vi "wrap.GetNameList.vi"(0 "class.GLue in":refnum<class "class.GLue.lvclass">, 5 "length":i32, 9 "index":i32=-1, 11 "error in (no error)":errorcluster, 13 "StringArray in":string[][](array[string])) -> (4 "class.GLue out":refnum<class "class.GLue.lvclass">, 6 "StringArray out":string[][](array[string]), 10 "return":i32, 15 "error out":errorcluster)   [LabVIEW 2014, in "GLue.lvlib" / "class.GLue.lvclass"]
uses:
  class.GLue.lvclass
  class.GLue.lvclass/class.GLue.ctl
  Resources/GLue.dll
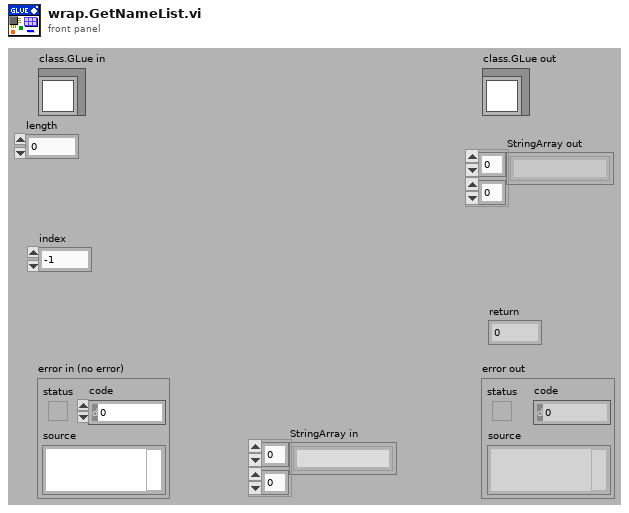
[diagram p1: front panel]
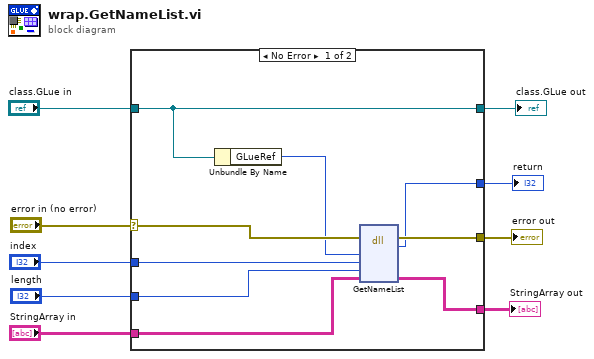
[diagram p0: block diagram]
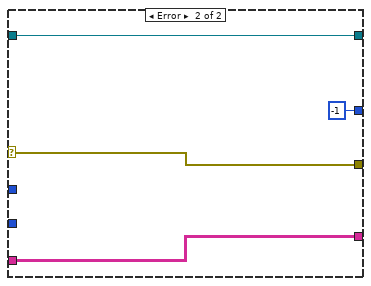
[diagram p2: hidden frame]
diagram:
  n1 = case shown="No Error" "error in (no error)" {
    selector: "error in (no error)" -> [w17 w22]
    tunnel: [w16 w22] -> w8
    tunnel: [w18 w21] -> w6
    tunnel: "class.GLue in" -> [w18 w21]
    tunnel: [w14 w20] -> w4
    tunnel: "StringArray in" -> [w13 w20]
    tunnel: "index" -> [w12 _]
    tunnel: [w11 -1 ("return")] -> w2
    tunnel: "length" -> [w10 _]
    frame No Error {
      n2 = Unbundle By Name(w18) -> ("GLueRef"=w15:i64)
      n3 = dll-call lib="C:/Users/Antonie/Documents/work/glue/trunk/Resources/GLue.dll" fn="GetNameList"(error in=w17, "MLua"=w15, "index"=w12, "length"=w10, "StringArray"=w13) -> (error out=w16:errorcluster, "return"=w11:i32, "StringArray"=w14:string[][])  [unwired: 5 in, 1 out]
    }
    frame Error {
    }
  }
  "error out" <- w8
  "class.GLue out" <- w6
  "StringArray out" <- w4
  "return" <- w2
